vi "log analysis_gps.vi"() -> ()   [LabVIEW 2018] (continued)
\t0.279000\t0.031000\n\t\n15:35:17.6\tlog_raw\tgps_raw\t#DUALANTENNAHEADINGA,USB3,0,49.5,FINESTEERING,2107,282935.600,02000000,d426,15824;INSUFFICIENT_OBS,NONE,-1.000000000,0.000000000,0.000000000,0.0,0.000000000,0.000000000,\"631T\",15,2,2,2,04,00,20,00*646f005d\n\tsystem status\tnormal 2 28.000000 0 0\trobot status\t256.780314\t90.298273\t8.714600\t-0.760632\t-2.225127\t150.467339\t0.388000\t-0.122000\n\t\n15:35:18.1\tlog_raw\tgps_raw\t#DUALANTENNAHEADINGA,USB3,0,49.5,FINESTEERING,2107,282936.100,02000000,d426,15824;INSUFFICIENT_OBS,NONE,-1.000000000,0.000000000,0.000000000,0.0,0.000000000,0.000000000,\"631T\",15,2,2,2,04,00,20,00*1eaf17a0\n\tsystem status\tnormal 2 27.900000 0 0\trobot status\t256.663990\t90.379029\t8.710300\t-0.683394\t-2.214514\t150.522988\t0.256000\t0.072000\n\t\n15:35:18.6\tlog_raw\tgps_raw\t#DUALANTENNAHEADINGA,USB3,0,49.5,FINESTEERING,2107,282936.600,02000000,d426,15824;INSUFFICIENT_OBS,NONE,-1.000000000,0.000000000,0.000000000,0.0,0.000000000,0.000000000,\"631T\",15,2,2,2,04,00,20,00*d2070d36\n\tsystem status\tnormal 2 28.000000 0 0\trobot status\t256.545030\t90.462138\t8.705100\t-0.490639\t-2.202791\t150.542142\t0.254000\t0.061000\n\t\n15:35:19.1\tlog_raw\tgps_raw\t#DUALANTENNAHEADINGA,USB3,0,49.5,FINESTEERING,2107,282937.100,02000000,d426,15824;INSUFFICIENT_OBS,NONE,-1.000000000,0.000000000,0.000000000,0.0,0.000000000,0.000000000,\"631T\",15,2,2,2,04,00,20,00*73771379\n\tsystem status\tnormal 2 27.900000 0 0\trobot status\t256.425827\t90.542953\t8.700000\t-0.567939\t-2.228448\t150.645686\t0.243000\t0.082000\n\t\n15:35:19.6\tlog_raw\tgps_raw\t#DUALANTENNAHEADINGA,USB3,0,50.0,FINESTEERING,2107,282937.600,02000000,d426,15824;INSUFFICIENT_OBS,NONE,-1.000000000,0.000000000,0.000000000,0.0,0.000000000,0.000000000,\"631T\",16,2,2,2,04,00,20,00*68ac25ab\n\tsystem status\tnormal 2 27.900000 0 0\trobot status\t256.306306\t90.622871\t8.696700\t-0.661354\t-2.128158\t150.731139\t0.241000\t0.099000\n\t\n15:35:20.1\tlog_raw\tgps_raw\t#DUALANTENNAHEADINGA,USB3,0,50.0,FINESTEERING,2107,282938.100,02000000,d426,15824;INSUFFICIENT_OBS,NONE,-1.000000000,0.000000000,0.000000000,0.0,0.000000000,0.000000000,\"631T\",16,2,2,2,04,00,20,00*a65f0d39\n\tsystem status\tnormal 2 27.900000 0 0\trobot status\t256.186382\t90.704627\t8.692700\t-0.606127\t-2.269498\t150.834524\t0.254000\t0.081000\n\t\n15:35:20.6\tlog_raw\tgps_raw\t#DUALANTENNAHEADINGA,USB3,0,50.0,FINESTEERING,2107,282938.600,02000000,d426,15824;INSUFFICIENT_OBS,NONE,-1.000000000,0.000000000,0.000000000,0.0,0.000000000,0.000000000,\"631T\",17,2,2,2,04,00,20,00*bd1597f7\n\tsystem status\tnormal 2 27.900000 0 0\trobot status\t256.067025\t90.786079\t8.688900\t-0.322241\t-2.499892\t151.028878\t0.352000\t-0.085000\n\t\n15:35:21.1\tlog_raw\tgps_raw\t#DUALANTENNAHEADINGA,USB3,0,50.0,FINESTEERING,2107,282939.100,02000000,d426,15824;INSUFFICIENT_OBS,NONE,-1.000000000,0.000000000,0.000000000,0.0,0.000000000,0.000000000,\"631T\",17,2,2,2,04,00,20,00*1c6589b8\n\tsystem status\tnormal 2 28.000000 0 0\trobot status\t255.947562\t90.865503\t8.685500\t-0.303833\t-2.363936\t151.114565\t0.300000\t0.000000\n\t\n15:35:21.6\tlog_raw\tgps_raw\t#DUALANTENNAHEADINGA,USB3,0,52.0,FINESTEERING,2107,282939.600,02000000,d426,15824;INSUFFICIENT_OBS,NONE,-1.000000000,0.000000000,0.000000000,0.0,0.000000000,0.000000000,\"631T\",14,2,2,2,04,00,20,00*bb12b8cf\n\tsystem status\tnormal 2 27.900000 0 0\trobot status\t255.828620\t90.941630\t8.682600\t-0.556904\t-2.247705\t151.117171\t0.272000\t0.029000\n\t\n15:35:22.1\tlog_raw\tgps_raw\t#DUALANTENNAHEADINGA,USB3,0,50.0,FINESTEERING,2107,282940.100,02000000,d426,15824;INSUFFICIENT_OBS,NONE,-1.000000000,0.000000000,0.000000000,0.0,0.000000000,0.000000000,\"631T\",14,2,2,2,04,00,20,00*9b77340d\n\tsystem status\tnormal 2 27.900000 0 0\trobot status\t255.707606\t91.021162\t8.679300\t-0.530900\t-2.252938\t151.145444\t0.328000\t-0.057000\n\t\n15:35:22.6\tlog_raw\tgps_raw\t#INSPVAXA,USB3,0,50.0,FINESTEERING,2107,282940.600,02000000,471d,15824;INS_ALIGNMENT_COMPLETE,INS_RTKFIXED,37.37095109367,126.72372052515,8.6731,22.3000,0.1517,-0.2300,-0.0234,-0.267173329,-2.329530247,298.720230899,0.4406,0.2945,0.5541,0.1133,0.0925,0.0773,0.0978,0.1028,4.9197,0f000001,0*f2292127\n\tsystem status\tnormal 2 28.000000 0 0\trobot status\t255.585782\t91.103037\t8.673100\t-0.267173\t-2.329530\t151.279769\t0.419000\t-0.188000\n\t\n15:35:23.1\tlog_raw\tgps_raw\t#DUALANTENNAHEADINGA,USB3,0,49.5,FINESTEERING,2107,282941.100,02000000,d426,15824;INSUFFICIENT_OBS,NONE,-1.000000000,0.000000000,0.000000000,0.0,0.000000000,0.000000000,\"631T\",17,2,2,2,04,00,20,00*21dc1c90\n\tsystem status\tnormal 2 28.000000 0 0\trobot status\t255.466813\t91.182906\t8.667600\t-0.154589\t-2.350516\t151.330010\t0.342000\t-0.053000\n\t\n15:35:23.6\tlog_raw\tgps_raw\t#DUALANTENNAHEADINGA,USB3,0,49.5,FINESTEERING,2107,282941.600,02000000,d426,15824;INSUFFICIENT_OBS,NONE,-1.000000000,0.000000000,0.000000000,0.0,0.000000000,0.000000000,\"631T\",17,2,2,2,04,00,20,00*ed740606\n\tsystem status\tnormal 2 28.000000 0 0\trobot status\t255.348341\t91.260716\t8.663400\t-0.359685\t-2.297097\t151.358113\t0.271000\t0.037000\n\t\n15:35:24.1\tlog_raw\tgps_raw\t#DUALANTENNAHEADINGA,USB3,0,49.5,FINESTEERING,2107,282942.100,02000000,d426,15824;INSUFFICIENT_OBS,NONE,-1.000000000,0.000000000,0.000000000,0.0,0.000000000,0.000000000,\"631T\",15,2,2,2,04,00,20,00*e300170a\n\tsystem status\tnormal 2 27.900000 0 0\trobot status\t255.227088\t91.341470\t8.659200\t-0.418788\t-2.494250\t151.398248\t0.269000\t0.061000\n\t\n15:35:24.6\tlog_raw\tgps_raw\t#DUALANTENNAHEADINGA,USB3,0,49.5,FINESTEERING,2107,282942.600,02000000,d426,15824;INSUFFICIENT_OBS,NONE,-1.000000000,0.000000000,0.000000000,0.0,0.000000000,0.000000000,\"631T\",13,2,2,2,04,00,20,00*b274068f\n\tsystem status\tnormal 2 28.000000 0 0\trobot status\t255.107667\t91.421781\t8.652400\t-0.280884\t-2.457147\t151.424820\t0.260000\t0.059000\n\t\n15:35:25.1\tlog_raw\tgps_raw\t#DUALANTENNAHEADINGA,USB3,0,49.5,FINESTEERING,2107,282943.100,02008000,d426,15824;INSUFFICIENT_OBS,NONE,-1.000000000,0.000000000,0.000000000,0.0,0.000000000,0.000000000,\"631T\",13,2,2,2,04,00,20,00*05979c61\n\tsystem status\tnormal 2 28.000000 0 0\trobot status\t254.990314\t91.500800\t8.645200\t-0.235303\t-2.314324\t151.467138\t0.287000\t0.019000\n\t\n15:35:25.6\tlog_raw\tgps_raw\t#DUALANTENNAHEADINGA,USB3,0,50.0,FINESTEERING,2107,282943.600,02008000,d426,15824;INSUFFICIENT_OBS,NONE,-1.000000000,0.000000000,0.000000000,0.0,0.000000000,0.000000000,\"631T\",15,2,2,2,04,00,20,00*20c62709\n\tsystem status\tnormal 2 28.000000 0 0\trobot status\t254.870895\t91.580665\t8.639100\t-0.192889\t-2.377459\t151.460910\t0.281000\t0.026000\n\t\n15:35:26.1\tlog_raw\tgps_raw\t#DUALANTENNAHEADINGA,USB3,0,50.0,FINESTEERING,2107,282944.100,02008000,d426,15824;INSUFFICIENT_OBS,NONE,-1.000000000,0.000000000,0.000000000,0.0,0.000000000,0.000000000,\"631T\",15,2,2,2,04,00,20,00*361725d1\n\tsystem status\tnormal 2 28.000000 0 0\trobot status\t254.750757\t91.660864\t8.633300\t-0.180871\t-2.554639\t151.458844\t0.261000\t0.067000\n\t\n15:35:26.6\tlog_raw\tgps_raw\t#DUALANTENNAHEADINGA,USB3,0,53.0,FINESTEERING,2107,282944.600,02008000,d426,15824;INSUFFICIENT_OBS,NONE,-1.000000000,0.000000000,0.000000000,0.0,0.000000000,0.000000000,\"631T\",15,2,2,2,04,00,20,00*567244ab\n\tsystem status\tnormal 2 28.000000 0 0\trobot status\t254.630389\t91.742058\t8.625500\t-0.192952\t-2.590747\t151.439255\t0.283000\t0.030000\n\t\n15:35:27.1\tlog_raw\tgps_raw\t#DUALANTENNAHEADINGA,USB3,0,52.5,FINESTEERING,2107,282945.100,02008000,d426,15824;INSUFFICIENT_OBS,NONE,-1.000000000,0.000000000,0.000000000,0.0,0.000000000,0.000000000,\"631T\",13,2,2,2,04,00,20,00*5be0619f\n\tsystem status\tnormal 2 28.000000 0 0\trobot status\t254.513468\t91.822238\t8.617100\t-0.159086\t-2.547197\t151.443587\t0.276000\t0.035000\n\t\n15:35:27.6\tlog_raw\tgps_raw\t#DUALANTENNAHEADINGA,USB3,0,52.5,FINESTEERING,2107,282945.600,02008000,d426,15824;INSUFFICIENT_OBS,NONE,-1.000000000,0.000000000,0.000000000,0.0,0.000000000,0.000000000,\"631T\",13,2,2,2,04,00,20,00*97487b09\n\tsystem status\tnormal 2 28.000000 0 0\trobot status\t254.392942\t91.902806\t8.609000\t-0.121394\t-2.673746\t151.420849\t0.277000\t0.034000\n\t\n15:35:28.1\tlog_raw\tgps_raw\t#DUALANTENNAHEADINGA,USB3,0,49.5,FINESTEERING,2107,282946.100,02008000,d426,15824;INSUFFICIENT_OBS,NONE,-1.000000000,0.000000000,0.000000000,0.0,0.000000000,0.000000000,\"631T\",14,2,2,2,04,00,20,00*4e6006d6\n\tsystem status\tnormal 2 28.000000 0 0\trobot status\t254.275148\t91.981980\t8.600700\t-0.137266\t-2.581289\t151.414534\t0.312000\t-0.003000\n\t\n15:35:28.6\tlog_raw\tgps_raw\t#DUALANTENNAHEADINGA,USB3,0,49.5,FINESTEERING,2107,282946.600,02008000,d426,15824;INSUFFICIENT_OBS,NONE,-1.000000000,0.000000000,0.000000000,0.0,0.000000000,0.000000000,\"631T\",15,2,2,2,04,00,20,00*552a9c18\n\tsystem status\tnormal 2 28.000000 0 0\trobot status\t254.158680\t92.060277\t8.593000\t-0.236334\t-2.525811\t151.415418\t0.436000\t-0.193000\n\t\n15:35:29.1\tlog_raw\tgps_raw\t#DUALANTENNAHEADINGA,USB3,0,48.5,FINESTEERING,2107,282947.100,02008000,d426,15824;INSUFFICIENT_OBS,NONE,-1.000000000,0.000000000,0.000000000,0.0,0.000000000,0.000000000,\"631T\",16,2,2,2,04,00,20,00*3348d25a\n\tsystem status\tnormal 2 28.000000 0 0\trobot status\t254.042373\t92.139923\t8.584700\t-0.240278\t-2.555508\t151.434704\t0.283000\t0.033000\n\t\n15:35:29.6\tlog_raw\tgps_raw\t#DUALANTENNAHEADINGA,USB3,0,48.5,FINESTEERING,2107,282947.600,02000000,d426,15824;INSUFFICIENT_OBS,NONE,-1.000000000,0.000000000,0.000000000,0.0,0.000000000,0.000000000,\"631T\",16,2,2,2,04,00,20,00*e9734c6d\n\tsystem status\tnormal 2 27.900000 0 0\trobot status\t253.922648\t92.221882\t8.576200\t-0.258547\t-2.691459\t151.424743\t0.237000\t0.095000\n\t\n15:35:30.1\tlog_raw\tgps_raw\t#DUALANTENNAHEADINGA,USB3,0,48.5,FINESTEERING,2107,282948.100,02000000,d426,15824;INSUFFICIENT_OBS,NONE,-1.000000000,0.000000000,0.000000000,0.0,0.000000000,0.000000000,\"631T\",16,2,2,2,04,00,20,00*278064ff\n\tsystem status\tnormal 2 28.000000 0 0\trobot status\t253.805920\t92.302649\t8.568900\t-0.289763\t-2.670093\t151.392243\t0.351000\t-0.076000\n\t\n15:35:30.6\tlog_raw\tgps_raw\t#DUALANTENNAHEADINGA,USB3,0,49.0,FINESTEERING,2107,282948.600,02000000,d426,15824;INSUFFICIENT_OBS,NONE,-1.000000000,0.000000000,0.000000000,0.0,0.000000000,0.000000000,\"631T\",16,2,2,2,04,00,20,00*da164e01\n\tsystem status\tnormal 2 28.000000 0 0\trobot status\t253.687845\t92.382279\t8.561200\t-0.417432\t-2.808123\t151.452850\t0.423000\t-0.185000\n\t\n15:35:31.1\tlog_raw\tgps_raw\t#DUALANTENNAHEADINGA,USB3,0,49.0,FINESTEERING,2107,282949.100,02008000,d426,15824;INSUFFICIENT_OBS,NONE,-1.000000000,0.000000000,0.000000000,0.0,0.000000000,0.000000000,\"631T\",16,2,2,2,04,00,20,00*6df5d4ef\n\tsystem status\tnormal 2 27.900000 0 0\trobot status\t253.568870\t92.461854\t8.552900\t-0.517935\t-2.852279\t151.503432\t0.247000\t0.081000\n\t\n15:35:31.6\tlog_raw\tgps_raw\t#DUALANTENNAHEADINGA,USB3,0,50.5,FINESTEERING,2107,282949.600,02008000,d426,15824;INSUFFICIENT_OBS,NONE,-1.000000000,0.000000000,0.000000000,0.0,0.000000000,0.000000000,\"631T\",16,2,2,2,04,00,20,00*d5786494\n\tsystem status\tnormal 2 27.900000 0 0\trobot status\t253.447549\t92.540563\t8.545300\t-0.634770\t-2.802068\t151.569225\t0.458000\t-0.230000\n\t\n15:35:32.1\tlog_raw\tgps_raw\t#DUALANTENNAHEADINGA,USB3,0,50.5,FINESTEERING,2107,282950.100,02008000,d426,15824;INSUFFICIENT_OBS,NONE,-1.000000000,0.000000000,0.000000000,0.0,0.000000000,0.000000000,\"631T\",16,2,2,2,04,00,20,00*5348e2e5\n\tsystem status\tnormal 2 28.000000 0 0\trobot status\t253.327603\t92.619270\t8.538000\t-0.695995\t-2.872123\t151.658329\t0.256000\t0.081000\n\t\n15:35:32.6\tlog_raw\tgps_raw\t#DUALANTENNAHEADINGA,USB3,0,50.5,FINESTEERING,2107,282950.600,02008000,d426,15824;INSUFFICIENT_OBS,NONE,-1.000000000,0.000000000,0.000000000,0.0,0.000000000,0.000000000,\"631T\",16,2,2,2,04,00,20,00*9fe0f873\n\tsystem status\tnormal 2 27.900000 0 0\trobot status\t253.206959\t92.699516\t8.530600\t-0.579326\t-2.998121\t151.745125\t0.276000\t0.032000\n\t\n15:35:33.1\tlog_raw\tgps_raw\t#DUALANTENNAHEADINGA,USB3,0,48.0,FINESTEERING,2107,282951.100,02008000,d426,15824;INSUFFICIENT_OBS,NONE,-1.000000000,0.000000000,0.000000000,0.0,0.000000000,0.000000000,\"631T\",16,2,2,2,04,00,20,00*2ef19a75\n\tsystem status\tnormal 2 27.900000 0 0\trobot status\t253.086641\t92.778208\t8.522800\t-0.669072\t-2.968137\t151.793358\t0.305000\t-0.020000\n\t\n15:35:33.6\tlog_raw\tgps_raw\t#DUALANTENNAHEADINGA,USB3,0,48.0,FINESTEERING,2107,282951.600,02008000,d426,15824;INSUFFICIENT_OBS,NONE,-1.000000000,0.000000000,0.000000000,0.0,0.000000000,0.000000000,\"631T\",17,2,2,2,04,00,20,00*35bb00bb\n\tsystem status\tnormal 2 28.000000 0 0\trobot status\t252.966146\t92.856684\t8.515700\t-0.823336\t-2.969880\t151.842849\t0.277000\t0.026000\n\t\n15:35:34.1\tlog_raw\tgps_raw\t\tsystem status\tnormal 2 27.900000 0 0\trobot status\t252.845707\t92.935485\t8.508700\t-0.946775\t-3.084704\t151.928566\t0.199000\t0.137000\n\t\n15:35:34.6\tlog_raw\tgps_raw\t\tsystem status\tnormal 2 28.000000 0 0\trobot status\t252.727118\t93.014271\t8.504100\t-0.880224\t-2.934570\t152.110413\t0.448000\t-0.238000\n\t\n15:35:35.1\tlog_raw\tgps_raw\t#DUALANTENNAHEADINGA,USB3,0,47.5,FINESTEERING,2107,282953.100,02008000,d426,15824;INSUFFICIENT_OBS,NONE,-1.000000000,0.000000000,0.000000000,0.0,0.000000000,0.000000000,\"631T\",14,2,2,2,04,00,20,00*a6e4ed65\n\tsystem status\tnormal 2 27.900000 0 0\trobot status\t252.606768\t93.093325\t8.499800\t-0.892042\t-2.837254\t152.160427\t0.275000\t0.033000\n\t\n15:35:35.6\tlog_raw\tgps_raw\t#DUALANTENNAHEADINGA,USB3,0,50.0,FINESTEERING,2107,282953.600,02000000,d426,15824;INSUFFICIENT_OBS,NONE,-1.000000000,0.000000000,0.000000000,0.0,0.000000000,0.000000000,\"631T\",13,2,2,2,04,00,20,00*54eb1acf\n\tsystem status\tnormal 2 27.900000 0 0\trobot status\t252.486962\t93.170128\t8.495600\t-0.968428\t-2.739285\t152.198894\t0.348000\t-0.080000\n\t\n15:35:36.1\tlog_raw\tgps_raw\t#DUALANTENNAHEADINGA,USB3,0,48.0,FINESTEERING,2107,282954.100,02000000,d426,15824;INSUFFICIENT_OBS,NONE,-1.000000000,0.000000000,0.000000000,0.0,0.000000000,0.000000000,\"631T\",14,2,2,2,04,00,20,00*4d1f09d9\n\tsystem status\tnormal 2 27.900000 0 0\trobot status\t252.367322\t93.248054\t8.491100\t-0.955023\t-2.515838\t152.247418\t0.357000\t-0.086000\n\t\n15:35:36.6\tlog_raw\tgps_raw\t#DUALANTENNAHEADINGA,USB3,0,48.0,FINESTEERING,2107,282954.600,02000000,d426,15824;INSUFFICIENT_OBS,NONE,-1.000000000,0.000000000,0.000000000,0.0,0.000000000,0.000000000,\"631T\",16,2,2,2,04,00,20,00*f50315be\n\tsystem status\tnormal 2 28.000000 0 0\trobot status\t252.247855\t93.326149\t8.487100\t-0.842888\t-2.348222\t152.261330\t0.322000\t-0.041000\n\t\n15:35:37.1\tlog_raw\tgps_raw\t#INSPVAXA,USB3,0,47.5,FINESTEERING,2107,282955.150,02000000,471d,15824;INS_ALIGNMENT_COMPLETE,INS_RTKFIXED,37.37097191028,126.72368135449,8.4841,22.3000,0.1693,-0.2422,-0.0142,-0.799407397,-2.166438439,297.747094152,0.4450,0.2953,0.5584,0.1141,0.0928,0.0775,0.0978,0.1030,4.9299,0f000001,0*711ec271\n\tsystem status\tnormal 2 28.000000 0 0\trobot status\t252.116109\t93.413465\t8.484100\t-0.799407\t-2.166438\t152.252906\t0.332000\t-0.052000\n\t\n15:35:37.6\tlog_raw\tgps_raw\t#DUALANTENNAHEADINGA,USB3,0,47.5,FINESTEERING,2107,282955.600,02000000,d426,15824;INSUFFICIENT_OBS,NONE,-1.000000000,0.000000000,0.000000000,0.0,0.000000000,0.000000000,\"631T\",13,2,2,2,04,00,20,00*8140e48e\n\tsystem status\tnormal 2 27.900000 0 0\trobot status\t252.011078\t93.483113\t8.481000\t-0.846538\t-1.955023\t152.315960\t0.339000\t-0.062000\n\t\n15:35:38.1\tlog_raw\tgps_raw\t#DUALANTENNAHEADINGA,USB3,0,47.5,FINESTEERING,2107,282956.100,02000000,d426,15824;INSUFFICIENT_OBS,NONE,-1.000000000,0.000000000,0.000000000,0.0,0.000000000,0.000000000,\"631T\",14,2,2,2,04,00,20,00*b1be7838\n\tsystem status\tnormal 2 27.900000 0 0\trobot status\t251.892792\t93.560878\t8.478700\t-1.086649\t-1.737827\t152.384884\t0.296000\t-0.002000\n\t\n15:35:38.6\tlog_raw\tgps_raw\t\tsystem status\tnormal 2 28.000000 0 0\trobot status\t251.773181\t93.640986\t8.476600\t-0.964983\t-1.456887\t152.427884\t0.357000\t-0.090000\n\t\n15:35:39.1\tlog_raw\tgps_raw\t#DUALANTENNAHEADINGA,USB3,0,49.5,FINESTEERING,2107,282957.100,02000000,d426,15824;INSUFFICIENT_OBS,NONE,-1.000000000,0.000000000,0.000000000,0.0,0.000000000,0.000000000,\"631T\",15,2,2,2,04,00,20,00*1dabb482\n\tsystem status\tnormal 2 28.000000 0 0\trobot status\t251.654659\t93.722946\t8.475100\t-0.668177\t-1.430088\t152.409420\t0.366000\t-0.112000\n\t\n15:35:39.6\tlog_raw\tgps_raw\t\tsystem status\tnormal 2 28.000000 0 0\trobot status\t251.542323\t93.800199\t8.475200\t-0.574923\t-1.096038\t152.514245\t0.289000\t-0.013000\n\t\n15:35:40.1\tlog_raw\tgps_raw\t#DUALANTENNAHEADINGA,USB3,0,47.5,FINESTEERING,2107,282958.100,02000000,d426,15824;INSUFFICIENT_OBS,NONE,-1.000000000,0.000000000,0.000000000,0.0,0.000000000,0.000000000,\"631T\",14,2,2,2,04,00,20,00*de3d4ee5\n\tsystem status\tnormal 2 28.000000 0 0\trobot status\t251.415981\t93.883006\t8.474100\t-0.824722\t-1.034335\t152.447929\t0.230000\t0.080000\n\t\n15:35:40.6\tlog_raw\tgps_raw\t#DUALANTENNAHEADINGA,USB3,0,47.5,FINESTEERING,2107,282958.600,02000000,d426,15824;INSUFFICIENT_OBS,NONE,-1.000000000,0.000000000,0.000000000,0.0,0.000000000,0.000000000,\"631T\",15,2,2,2,04,00,20,00*c577d42b\n\tsystem status\tnormal 2 28.000000 0 0\trobot status\t251.291310\t93.963969\t8.471000\t-1.101436\t-1.443310\t152.459219\t0.236000\t0.098000\n\t\n15:35:41.1\tlog_raw\tgps_raw\t#DUALANTENNAHEADINGA,USB3,0,47.5,FINESTEERING,2107,282959.100,02000000,d426,15824;INSUFFICIENT_OBS,NONE,-1.000000000,0.000000000,0.000000000,0.0,0.000000000,0.000000000,\"631T\",15,2,2,2,04,00,20,00*6407ca64\n\tsystem status\tnormal 2 28.000000 0 0\trobot status\t251.172018\t94.044368\t8.468600\t-1.020791\t-1.480021\t152.538410\t0.271000\t0.040000\n\t\n15:35:41.6\tlog_raw\tgps_raw\t#INSPVAXA,USB3,0,50.5,FINESTEERING,2107,282959.650,02000000,471d,15824;INS_ALIGNMENT_COMPLETE,INS_RTKFIXED,37.37097835365,126.72366921356,8.4679,22.3000,0.1677,-0.2288,-0.0117,-1.228660842,-1.304176220,297.349897082,0.4459,0.2954,0.5577,0.1140,0.0926,0.0775,0.0977,0.1029,4.9210,0f000001,0*0060fe10\n\tsystem status\tnormal 2 27.900000 0 0\trobot status\t251.040686\t94.128612\t8.467900\t-1.228661\t-1.304176\t152.650103\t0.294000\t0.025000\n\t\n15:35:42.1\tlog_raw\tgps_raw\t#DUALANTENNAHEADINGA,USB3,0,50.5,FINESTEERING,2107,282960.100,02000000,d426,15824;INSUFFICIENT_OBS,NONE,-1.000000000,0.000000000,0.000000000,0.0,0.000000000,0.000000000,\"631T\",15,2,2,2,04,00,20,00*3c5b3030\n\tsystem status\tnormal 2 27.900000 0 0\trobot status\t250.933323\t94.199664\t8.470400\t-1.218748\t-1.601096\t152.690711\t0.293000\t0.046000\n\t\n15:35:42.6\tlog_raw\tgps_raw\t#INSPVAXA,USB3,0,51.0,FINESTEERING,2107,282960.650,02000000,471d,15824;INS_ALIGNMENT_COMPLETE,INS_RTKFIXED,37.37097975694,126.72366653039,8.4696,22.3000,0.1798,-0.2500,-0.0237,-1.216813697,-1.020291327,297.186745647,0.4456,0.2953,0.5575,0.1139,0.0925,0.0775,0.0977,0.1029,4.9186,0f000001,0*5a2daee3\n\tsystem status\tnormal 2 27.900000 0 0\trobot status\t250.803015\t94.284363\t8.469600\t-1.216814\t-1.020291\t152.813254\t0.376000\t-0.091000\n\t\n15:35:43.1\tlog_raw\tgps_raw\t#INSPVAXA,USB3,0,49.5,FINESTEERING,2107,282961.150,02000000,471d,15824;INS_ALIGNMENT_COMPLETE,INS_RTKFIXED,37.37098043030,126.72366522949,8.4707,22.3000,0.1736,-0.2321,-0.0202,-1.283284978,-0.599057557,297.054686065,0.4445,0.2952,0.5571,0.1143,0.0927,0.0774,0.0977,0.1029,4.9180,0f000001,0*2a0011a7\n\tsystem status\tnormal 2 27.900000 0 0\trobot status\t250.687783\t94.359099\t8.470700\t-1.283285\t-0.599058\t152.945314\t0.285000\t0.038000\n\t\n15:35:43.6\tlog_raw\tgps_raw\t#INSPVAXA,USB3,0,49.5,FINESTEERING,2107,282961.650,02000000,471d,15824;INS_ALIGNMENT_COMPLETE,INS_RTKFIXED,37.37098110598,126.72366388035,8.4719,22.3000,0.1770,-0.2280,-0.0121,-1.256734813,-0.468526874,296.976116975,0.4445,0.2952,0.5571,0.1143,0.0927,0.0774,0.0977,0.1029,4.9180,0f000001,0*1df4362b\n\tsystem status\tnormal 2 27.900000 0 0\trobot status\t250.568279\t94.434093\t8.471900\t-1.256735\t-0.468527\t153.023883\t0.258000\t0.074000\n\t\n15:35:44.1\tlog_raw\tgps_raw\t\tsystem status\tnormal 2 27.900000 0 0\trobot status\t250.460513\t94.502707\t8.473000\t-1.216741\t-0.450959\t153.062982\t0.253000\t0.073000\n\t\n15:35:44.6\tlog_raw\tgps_raw\t#INSPVAXA,USB3,0,47.5,FINESTEERING,2107,282962.650,02000000,471d,15824;INS_ALIGNMENT_COMPLETE,INS_RTKFIXED,37.37098248042,126.72366115831,8.4743,22.3000,0.1748,-0.2259,-0.0058,-1.109471355,-0.449070026,296.783460113,0.4449,0.2952,0.5570,0.1145,0.0926,0.0774,0.0977,0.1028,4.9165,0f000001,0*1baf4086\n\tsystem status\tnormal 2 27.900000 0 0\trobot status\t250.327165\t94.586642\t8.474300\t-1.109471\t-0.449070\t153.216540\t0.253000\t0.063000\n\t\n15:35:45.1\tlog_raw\tgps_raw\t#INSPVAXA,USB3,0,50.0,FINESTEERING,2107,282963.150,02000000,471d,15824;INS_ALIGNMENT_COMPLETE,INS_RTKFIXED,37.37098316293,126.72365977185,8.4754,22.3000,0.1768,-0.2291,-0.0058,-1.166384904,-0.522599748,296.670399904,0.4455,0.2951,0.5568,0.1141,0.0925,0.0774,0.0977,0.1028,4.9146,0f000001,0*0f185e23\n\tsystem status\tnormal 2 27.900000 0 0\trobot status\t250.204354\t94.662394\t8.475400\t-1.166385\t-0.522600\t153.329600\t0.333000\t-0.037000\n\t\n15:35:45.6\tlog_raw\tgps_raw\t#INSPVAXA,USB3,0,50.0,FINESTEERING,2107,282963.650,02000000,471d,15824;INS_ALIGNMENT_COMPLETE,INS_RTKFIXED,37.37098384842,126.72365839732,8.4765,22.3000,0.1700,-0.2283,-0.0073,-1.035044239,-0.558854853,296.631402056,0.4455,0.2951,0.5568,0.1141,0.0925,0.0774,0.0977,0.1028,4.9146,0f000001,0*d0797a7e\n\tsystem status\tnormal 2 27.900000 0 0\trobot status\t250.082601\t94.738476\t8.476500\t-1.035044\t-0.558855\t153.368598\t0.256000\t0.071000\n\t\n15:35:46.1\tlog_raw\tgps_raw\t#INSPVAXA,USB3,0,47.5,FINESTEERING,2107,282964.150,02000000,471d,15824;INS_ALIGNMENT_COMPLETE,INS_RTKFIXED,37.37098452995,126.72365703977,8.4774,22.3000,0.1687,-0.2278,-0.0051,-0.825749574,-0.403704202,296.577547873,0.4447,0.2949,0.5563,0.1141,0.0926,0.0774,0.0977,0.1028,4.9134,0f000001,0*96a6dd12\n\tsystem status\tnormal 2 28.000000 0 0\trobot status\t249.962351\t94.814119\t8.477400\t-0.825750\t-0.403704\t153.422452\t0.285000\t0.028000\n\t\n15:35:46.6\tlog_raw\tgps_raw\t#DUALANTENNAHEADINGA,USB3,0,47.5,FINESTEERING,2107,282964.600,02000000,d426,15824;INSUFFICIENT_OBS,NONE,-1.000000000,0.000000000,0.000000000,0.0,0.000000000,0.000000000,\"631T\",13,2,2,2,04,00,20,00*364e308a\n\tsystem status\tnormal 2 27.900000 0 0\trobot status\t249.853356\t94.880309\t8.477500\t-0.801435\t-0.341855\t153.481008\t0.370000\t-0.101000\n\t\n15:35:47.1\tlog_raw\tgps_raw\t#INSPVAXA,USB3,0,49.0,FINESTEERING,2107,282965.150,02000000,471d,15824;INS_ALIGNMENT_COMPLETE,INS_RTKFIXED,37.37098586278,126.72365430292,8.4776,22.3000,0.1652,-0.2280,-0.0084,-0.812912729,-0.298745474,296.545314243,0.4441,0.2948,0.5560,0.1139,0.0926,0.0774,0.0977,0.1027,4.9127,0f000001,0*10118c42\n\tsystem status\tnormal 2 28.000000 0 0\trobot status\t249.719925\t94.962050\t8.477600\t-0.812913\t-0.298745\t153.454686\t0.258000\t0.063000\n\t\n15:35:47.6\tlog_raw\tgps_raw\t#INSPVAXA,USB3,0,49.0,FINESTEERING,2107,282965.650,02000000,471d,15824;INS_ALIGNMENT_COMPLETE,INS_RTKFIXED,37.37098653582,126.72365294600,8.4789,22.3000,0.1677,-0.2410,-0.0069,-0.826772315,0.019774028,296.533621438,0.4441,0.2948,0.5560,0.1139,0.0926,0.0774,0.0977,0.1027,4.9127,0f000001,0*1d42ccbf\n\tsystem status\tnormal 2 28.000000 0 0\trobot status\t249.599732\t95.036751\t8.478900\t-0.826772\t0.019774\t153.466379\t0.367000\t-0.093000\n\t\n15:35:48.1\tlog_raw\tgps_raw\t\tsystem status\tnormal 2 27.900000 0 0\trobot status\t249.492164\t95.103838\t8.479600\t-0.859418\t0.051260\t153.510100\t0.350000\t-0.075000\n\t\n15:35:48.6\tlog_raw\tgps_raw\t\tsystem status\tnormal 2 28.000000 0 0\trobot status\t249.368260\t95.179421\t8.479400\t-0.924661\t-0.189774\t153.513644\t0.248000\t0.068000\n\t\n15:35:49.1\tlog_raw\tgps_raw\t#DUALANTENNAHEADINGA,USB3,0,48.5,FINESTEERING,2107,282967.100,02000000,d426,15824;INSUFFICIENT_OBS,NONE,-1.000000000,0.000000000,0.000000000,0.0,0.000000000,0.000000000,\"631T\",13,2,2,2,04,00,20,00*3ee5b9e8\n\tsystem status\tnormal 2 28.000000 0 0\trobot status\t249.246534\t95.255236\t8.479300\t-0.943512\t-0.176843\t153.495660\t0.260000\t0.060000\n\t\n15:35:49.6\tlog_raw\tgps_raw\t#INSPVAXA,USB3,0,48.5,FINESTEERING,2107,282967.650,02000000,471d,15824;INS_ALIGNMENT_COMPLETE,INS_RTKFIXED,37.37098925178,126.72364742874,8.4811,22.3000,0.1700,-0.2499,-0.0176,-0.986615151,-0.569191402,296.569428788,0.4450,0.2948,0.5562,0.1138,0.0925,0.0774,0.0977,0.1027,4.9114,0f000001,0*8120b203\n\tsystem status\tnormal 2 28.000000 0 0\trobot status\t249.111022\t95.338195\t8.481100\t-0.986615\t-0.569191\t153.430571\t0.300000\t0.000000\n\t\n15:35:50.1\tlog_raw\tgps_raw\t#INSPVAXA,USB3,0,51.0,FINESTEERING,2107,282968.150,02000000,471d,15824;INS_ALIGNMENT_COMPLETE,INS_RTKFIXED,37.37098994015,126.72364604242,8.4821,22.3000,0.1610,-0.2295,-0.0122,-1.022493310,-0.855866678,296.640582701,0.4448,0.2947,0.5563,0.1137,0.0927,0.0774,0.0977,0.1027,4.9112,0f000001,0*d8f4721a\n\tsystem status\tnormal 2 28.000000 0 0\trobot status\t248.988224\t95.414597\t8.482100\t-1.022493\t-0.855867\t153.359417\t0.284000\t0.007000\n\t\n15:35:50.6\tlog_raw\tgps_raw\t#INSPVAXA,USB3,0,51.0,FINESTEERING,2107,282968.650,02000000,471d,15824;INS_ALIGNMENT_COMPLETE,INS_RTKFIXED,37.37099061783,126.72364467060,8.4818,22.3000,0.1613,-0.2282,-0.0121,-1.153302728,-0.788505440,296.737399277,0.4448,0.2947,0.5563,0.1137,0.0927,0.0774,0.0977,0.1027,4.9112,0f000001,0*561016f0\n\tsystem status\tnormal 2 28.000000 0 0\trobot status\t248.866710\t95.489813\t8.481800\t-1.153303\t-0.788505\t153.262601\t0.294000\t0.000000\n\t\n15:35:51.1\tlog_raw\tgps_raw\t#INSPVAXA,USB3,0,51.0,FINESTEERING,2107,282969.150,02000000,471d,15824;INS_ALIGNMENT_COMPLETE,INS_RTKFIXED,37.37099130336,126.72364331886,8.4815,22.3000,0.1682,-0.2376,-0.0147,-1.125512606,-0.794604526,296.797111789,0.4434,0.2946,0.5560,0.1136,0.0926,0.0774,0.0977,0.1027,4.9114,0f000001,0*989702a1\n\tsystem status\tnormal 2 28.000000 0 0\trobot status\t248.746975\t95.565899\t8.481500\t-1.125513\t-0.794605\t153.202888\t0.298000\t-0.001000\n\t\n15:35:51.6\tlog_raw\tgps_raw\t#INSPVAXA,USB3,0,51.0,FINESTEERING,2107,282969.650,02000000,471d,15824;INS_ALIGNMENT_COMPLETE,INS_RTKFIXED,37.37099198077,126.72364195097,8.4825,22.3000,0.1618,-0.2351,-0.0139,-1.127841235,-0.916992124,296.845405459,0.4434,0.2946,0.5560,0.1136,0.0926,0.0774,0.0977,0.1027,4.9114,0f000001,0*282a9ea8\n\tsystem status\tnormal 2 28.000000 0 0\trobot status\t248.625810\t95.641085\t8.482500\t-1.127841\t-0.916992\t153.154595\t0.293000\t-0.005000\n\t\n15:35:52.1\tlog_raw\tgps_raw\t#INSPVAXA,USB3,0,49.5,FINESTEERING,2107,282970.150,02000000,471d,15824;INS_ALIGNMENT_COMPLETE,INS_RTKFIXED,37.37099263807,126.72364060691,8.4830,22.3000,0.1632,-0.2345,-0.0165,-1.327041845,-0.755974067,296.808985126,0.4427,0.2946,0.5559,0.1136,0.0925,0.0774,0.0977,0.1027,4.9120,0f000001,0*fb111f10\n\tsystem status\tnormal 2 28.000000 0 0\trobot status\t248.506755\t95.714039\t8.483000\t-1.327042\t-0.755974\t153.191015\t0.260000\t0.054000\n\t\n15:35:52.6\tlog_raw\tgps_raw\t#INSPVAXA,USB3,0,49.5,FINESTEERING,2107,282970.650,02000000,471d,15824;INS_ALIGNMENT_COMPLETE,INS_RTKFIXED,37.37099330542,126.72363923345,8.4843,22.3000,0.1650,-0.2334,-0.0103,-1.379297675,-0.666693531,296.810188523,0.4427,0.2946,0.5559,0.1136,0.0925,0.0774,0.0977,0.1027,4.9120,0f000001,0*40e7d89f\n\tsystem status\tnormal 2 28.000000 0 0\trobot status\t248.385097\t95.788108\t8.484300\t-1.379298\t-0.666694\t153.189811\t0.256000\t0.066000\n\t\n15:35:53.1\tlog_raw\tgps_raw\t#INSPVAXA,USB3,0,50.5,FINESTEERING,2107,282971.150,02000000,471d,15824;INS_ALIGNMENT_COMPLETE,INS_RTKFIXED,37.37099398804,126.72363786563,8.4853,22.3000,0.1661,-0.2338,-0.0180,-1.270685032,-0.682780948,296.817282496,0.4423,0.2946,0.5559,0.1136,0.0925,0.0774,0.0977,0.1027,4.9128,0f000001,0*f8a30bce\n\tsystem status\tnormal 2 27.900000 0 0\trobot status\t248.263937\t95.863872\t8.485300\t-1.270685\t-0.682781\t153.182718\t0.288000\t0.013000\n\t\n15:35:53.6\tlog_raw\tgps_raw\t#INSPVAXA,USB3,0,50.5,FINESTEERING,2107,282971.650,02000000,471d,15824;INS_ALIGNMENT_COMPLETE,INS_RTKFIXED,37.37099465990,126.72363651456,8.4846,22.3000,0.1699,-0.2362,-0.0068,-1.125018269,-0.570550984,296.760377501,0.4423,0.2946,0.5559,0.1136,0.0925,0.0774,0.0977,0.1027,4.9128,0f000001,0*ee20163a\n\tsystem status\tnormal 2 27.900000 0 0\trobot status\t248.144262\t95.938442\t8.484600\t-1.125018\t-0.570551\t153.239622\t0.292000\t0.006000\n\t\n15:35:54.1\tlog_raw\tgps_raw\t#INSPVAXA,USB3,0,48.5,FINESTEERING,2107,282972.150,02000000,471d,15824;INS_ALIGNMENT_COMPLETE,INS_RTKFIXED,37.37099533114,126.72363514569,8.4846,22.3000,0.1631,-0.2434,-0.0075,-1.229353207,-0.492392608,296.737479032,0.4422,0.2946,0.5560,0.1136,0.0925,0.0774,0.0977,0.1027,4.9138,0f000001,0*e2a3fa7c\n\tsystem status\tnormal 2 28.000000 0 0\trobot status\t248.035923\t96.005381\t8.484600\t-1.202885\t-0.495037\t153.210220\t0.342000\t-0.066000\n\t\n15:35:54.6\tlog_raw\tgps_raw\t#INSPVAXA,USB3,0,48.5,FINESTEERING,2107,282972.650,02000000,471d,15824;INS_ALIGNMENT_COMPLETE,INS_RTKFIXED,37.37099601296,126.72363373726,8.4848,22.3000,0.1655,-0.2434,-0.0062,-1.394785800,-0.542379073,296.812195855,0.4422,0.2946,0.5560,0.1136,0.0925,0.0774,0.0977,0.1027,4.9138,0f000001,0*ee63dd76\n\tsystem status\tnormal 2 28.000000 0 0\trobot status\t247.898253\t96.088618\t8.484800\t-1.394786\t-0.542379\t153.187804\t0.263000\t0.059000\n\t\n15:35:55.1\tlog_raw\tgps_raw\t#INSPVAXA,USB3,0,47.0,FINESTEERING,2107,282973.150,02000000,471d,15824;INS_ALIGNMENT_COMPLETE,INS_RTKFIXED,37.37099670386,126.72363233646,8.4846,22.3000,0.1605,-0.2379,-0.0037,-1.521129756,-0.763571260,296.778124874,0.4424,0.2946,0.5561,0.1137,0.0925,0.0774,0.0977,0.1027,4.9150,0f000001,0*6c9cf6ab\n\tsystem status\tnormal 2 28.000000 0 0\trobot status\t247.774172\t96.165301\t8.484600\t-1.521130\t-0.763571\t153.221875\t0.288000\t0.007000\n\t\n15:35:55.6\tlog_raw\tgps_raw\t#INSPVAXA,USB3,0,47.0,FINESTEERING,2107,282973.650,02000000,471d,15824;INS_ALIGNMENT_COMPLETE,INS_RTKFIXED,37.37099738989,126.72363093033,8.4852,22.3000,0.1673,-0.2327,0.0049,-1.602600322,-0.872352235,296.775722188,0.4424,0.2946,0.5561,0.1137,0.0925,0.0774,0.0977,0.1027,4.9150,0f000001,0*6d258e45\n\tsystem status\tnormal 2 27.900000 0 0\trobot status\t247.649620\t96.241443\t8.485200\t-1.602600\t-0.872352\t153.224278\t0.256000\t0.075000\n\t\n15:35:56.1\tlog_raw\tgps_raw\t\tsystem status\tnormal 2 27.900000 0 0\trobot status\t247.539986\t96.309557\t8.486500\t-1.695799\t-0.929134\t153.191391\t0.262000\t0.062000\n\t\n15:35:56.6\tlog_raw\tgps_raw\t#INSPVAXA,USB3,0,49.0,FINESTEERING,2107,282974.650,02000000,471d,15824;INS_ALIGNMENT_COMPLETE,INS_RTKFIXED,37.37099878397,126.72362813918,8.4887,22.3000,0.1782,-0.2307,0.0009,-1.519938045,-1.116202869,296.818721301,0.4416,0.2946,0.5560,0.1136,0.0925,0.0774,0.0977,0.1027,4.9163,0f000001,0*219b4438\n\tsystem status\tnormal 2 28.000000 0 0\trobot status\t247.402384\t96.396172\t8.488700\t-1.519938\t-1.116203\t153.181279\t0.376000\t-0.114000\n\t\n15:35:57.1\tlog_raw\tgps_raw\t#INSPVAXA,USB3,0,48.5,FINESTEERING,2107,282975.150,02000000,471d,15824;INS_ALIGNMENT_COMPLETE,INS_RTKFIXED,37.37099949137,126.72362674599,8.4896,22.3000,0.1736,-0.2362,0.0047,-1.445494984,-1.113340101,296.818619206,0.4431,0.2948,0.5567,0.1139,0.0926,0.0775,0.0977,0.1028,4.9177,0f000001,0*6f5d7051\n\tsystem status\tnormal 2 28.000000 0 0\trobot status\t247.278978\t96.474686\t8.489600\t-1.445495\t-1.113340\t153.181381\t0.296000\t0.021000\n\t\n15:35:57.6\tlog_raw\tgps_raw\t#INSPVAXA,USB3,0,48.5,FINESTEERING,2107,282975.650,02000000,471d,15824;INS_ALIGNMENT_COMPLETE,INS_RTKFIXED,37.37100019826,126.72362538278,8.4881,22.3000,0.1707,-0.2363,0.0005,-1.379938720,-0.916519890,296.842609438,0.4431,0.2948,0.5567,0.1139,0.0926,0.0775,0.0977,0.1028,4.9177,0f000001,0*5514ce87\n\tsystem status\tnormal 2 28.000000 0 0\trobot status\t247.158227\t96.553144\t8.488100\t-1.379939\t-0.916520\t153.157391\t0.250000\t0.083000\n\t\n15:35:58.1\tlog_raw\tgps_raw\t#INSPVAXA,USB3,0,49.5,FINESTEERING,2107,282976.150,02000000,471d,15824;INS_ALIGNMENT_COMPLETE,INS_RTKFIXED,37.37100091207,126.72362400101,8.4878,22.3000,0.1676,-0.2422,-0.0038,-1.345011262,-0.792526169,296.841980964,0.4425,0.2947,0.5567,0.1137,0.0926,0.0775,0.0977,0.1027,4.9188,0f000001,0*da02f91b\n\tsystem status\tnormal 2 27.900000 0 0\trobot status\t247.035832\t96.632369\t8.487800\t-1.345011\t-0.792526\t153.158019\t0.301000\t0.004000\n\t\n15:35:58.6\tlog_raw\tgps_raw\t#INSPVAXA,USB3,0,49.5,FINESTEERING,2107,282976.650,02000000,471d,15824;INS_ALIGNMENT_COMPLETE,INS_RTKFIXED,37.37100161787,126.72362259542,8.4876,22.3000,0.1713,-0.2361,-0.0000,-1.230290635,-0.956554131,296.705725068,0.4425,0.2947,0.5567,0.1137,0.0926,0.0775,0.0977,0.1027,4.9188,0f000001,0*8e2a3525\n\tsystem status\tnormal 2 27.900000 0 0\trobot status\t246.911327\t96.710706\t8.487600\t-1.230291\t-0.956554\t153.294275\t0.292000\t0.022000\n\t\n15:35:59.1\tlog_raw\tgps_raw\t#INSPVAXA,USB3,0,50.0,FINESTEERING,2107,282977.150,02000000,471d,15824;INS_ALIGNMENT_COMPLETE,INS_RTKFIXED,37.37100231261,126.72362121390,8.4877,22.3000,0.1651,-0.2421,0.0008,-1.098832221,-0.904742170,296.548603231,0.4420,0.2947,0.5566,0.1136,0.0926,0.0774,0.0977,0.1027,4.9199,0f000001,0*083bf95e\n\tsystem status\tnormal 2 27.900000 0 0\trobot status\t246.788954\t96.787815\t8.487700\t-1.098832\t-0.904742\t153.451397\t0.298000\t0.014000\n\t\n15:35:59.6\tlog_raw\tgps_raw\t#INSPVAXA,USB3,0,50.0,FINESTEERING,2107,282977.650,02000000,471d,15824;INS_ALIGNMENT_COMPLETE,INS_RTKFIXED,37.37100299121,126.72361981257,8.4879,22.3000,0.1659,-0.2302,-0.0060,-1.021895005,-0.933563278,296.461558193,0.4420,0.2947,0.5566,0.1136,0.0926,0.0774,0.0977,0.1027,4.9199,0f000001,0*f0f7e65a\n\tsystem status\tnormal 2 27.900000 0 0\trobot status\t246.664827\t96.863133\t8.487900\t-1.021895\t-0.933563\t153.538442\t0.283000\t0.028000\n\t\n15:36:00.1\tlog_raw\tgps_raw\t#INSPVAXA,USB3,0,52.0,FINESTEERING,2107,282978.150,02000000,471d,15824;INS_ALIGNMENT_COMPLETE,INS_RTKFIXED,37.37100367247,126.72361842907,8.4879,22.3000,0.1629,-0.2311,-0.0012,-0.920604944,-1.043526299,296.260165463,0.4427,0.2948,0.5570,0.1137,0.0928,0.0775,0.0977,0.1027,4.9208,0f000001,0*6c36e752\n\tsystem status\tnormal 2 27.900000 0 0\trobot status\t246.542279\t96.938746\t8.487900\t-0.920605\t-1.043526\t153.739835\t0.272000\t0.033000\n\t\n15:36:00.6\tlog_raw\tgps_raw\t#INSPVAXA,USB3,0,52.0,FINESTEERING,2107,282978.650,02000000,471d,15824;INS_ALIGNMENT_COMPLETE,INS_RTKFIXED,37.37100436684,126.72361701359,8.4867,22.3000,0.1639,-0.2335,-0.0162,-0.883856990,-1.214783963,296.168399886,0.4427,0.2948,0.5570,0.1137,0.0928,0.0775,0.0977,0.1027,4.9208,0f000001,0*f7bb67d2\n\tsystem status\tnormal 2 27.900000 0 0\trobot status\t246.416898\t97.015814\t8.486700\t-0.883857\t-1.214784\t153.831600\t0.370000\t-0.102000\n\t\n15:36:01.1\tlog_raw\tgps_raw\t#INSPVAXA,USB3,0,51.5,FINESTEERING,2107,282979.150,02000000,471d,15824;INS_ALIGNMENT_COMPLETE,INS_RTKFIXED,37.37100504962,126.72361562716,8.4847,22.3000,0.1600,-0.2330,-0.0182,-0.879226259,-1.131302419,296.112400832,0.4429,0.2948,0.5572,0.1137,0.0928,0.0775,0.0977,0.1027,4.9212,0f000001,0*44fc000f\n\tsystem status\tnormal 2 28.000000 0 0\trobot status\t246.294090\t97.091595\t8.484700\t-0.879226\t-1.131302\t153.887599\t0.432000\t-0.202000\n\t\n15:36:01.6\tlog_raw\tgps_raw\t\tsystem status\tnormal 2 27.900000 0 0\trobot status\t246.169041\t97.167187\t8.484100\t-0.926329\t-1.223584\t153.988143\t0.213000\t0.127000\n\t\n15:36:02.1\tlog_raw\tgps_raw\t#INSPVAXA,USB3,0,48.0,FINESTEERING,2107,282980.150,02000000,471d,15824;INS_ALIGNMENT_COMPLETE,INS_RTKFIXED,37.37100639827,126.72361280580,8.4843,22.3000,0.1610,-0.2464,-0.0078,-1.128808360,-1.315408116,295.882124797,0.4447,0.2950,0.5582,0.1140,0.0927,0.0775,0.0977,0.1028,4.9213,0f000001,0*5399c86c\n\tsystem status\tnormal 2 27.900000 0 0\trobot status\t246.044179\t97.241282\t8.484300\t-1.128808\t-1.315408\t154.117875\t0.355000\t-0.079000\n\t\n15:36:02.6\tlog_raw\tgps_raw\t#INSPVAXA,USB3,0,48.0,FINESTEERING,2107,282980.650,02000000,471d,15824;INS_ALIGNMENT_COMPLETE,INS_RTKFIXED,37.37100705164,126.72361137761,8.4834,22.3000,0.1707,-0.2402,-0.0119,-1.407160941,-1.329354223,295.708309677,0.4447,0.2950,0.5582,0.1140,0.0927,0.0775,0.0977,0.1028,4.9213,0f000001,0*d4834280\n\tsystem status\tnormal 2 27.900000 0 0\trobot status\t245.917672\t97.313800\t8.483400\t-1.407161\t-1.329354\t154.291690\t0.263000\t0.067000\n\t\n15:36:03.1\tlog_raw\tgps_raw\t#INSPVAXA,USB3,0,48.5,FINESTEERING,2107,282981.150,02000000,471d,15824;INS_ALIGNMENT_COMPLETE,INS_RTKFIXED,37.37100772173,126.72360998460,8.4814,22.3000,0.1860,-0.2371,-0.0157,-1.203417733,-1.261430362,295.578766556,0.4455,0.2951,0.5589,0.1141,0.0926,0.0776,0.0977,0.1028,4.9213,0f000001,0*2091f446\n\tsystem status\tnormal 2 27.900000 0 0\trobot status\t245.794281\t97.388173\t8.481400\t-1.203418\t-1.261430\t154.421233\t0.264000\t0.066000\n\t\n15:36:03.6\tlog_raw\tgps_raw\t\tsystem status\tnormal 2 27.900000 0 0\trobot status\t245.671083\t97.462988\t8.476500\t-0.879247\t-1.278490\t154.524074\t0.350000\t-0.056000\n\t\n15:36:04.1\tlog_raw\tgps_raw\t\tsystem status\tnormal 2 27.900000 0 0\trobot status\t245.548324\t97.535797\t8.471000\t-0.912734\t-1.315304\t154.588410\t0.258000\t0.074000\n\t\n15:36:04.6\tlog_raw\tgps_raw\t\tsystem status\tnormal 2 27.900000 0 0\trobot status\t245.424899\t97.608212\t8.466300\t-1.011673\t-1.263689\t154.596842\t0.326000\t-0.041000\n\t\n15:36:05.1\tlog_raw\tgps_raw\t#INSPVAXA,USB3,0,51.0,FINESTEERING,2107,282983.150,02000000,471d,15824;INS_ALIGNMENT_COMPLETE,INS_RTKFIXED,37.37101036366,126.72360442489,8.4628,22.3000,0.1755,-0.2357,-0.0080,-1.025739547,-1.189368406,295.388361945,0.4463,0.2951,0.5596,0.1141,0.0926,0.0776,0.0978,0.1028,4.9221,0f000001,0*2959208b\n\tsystem status\tnormal 2 27.900000 0 0\trobot status\t245.301811\t97.681401\t8.462800\t-1.025740\t-1.189368\t154.611638\t0.284000\t0.031000\n\t\n15:36:05.6\tlog_raw\tgps_raw\t#INSPVAXA,USB3,0,51.0,FINESTEERING,2107,282983.650,02000000,471d,15824;INS_ALIGNMENT_COMPLETE,INS_RTKFIXED,37.37101102324,126.72360304881,8.4600,22.3000,0.1712,-0.2258,-0.0116,-0.859579681,-1.039097489,295.288660935,0.4463,0.2951,0.5596,0.1141,0.0926,0.0776,0.0978,0.1028,4.9221,0f000001,0*ad7af1a9\n\tsystem status\tnormal 2 28.000000 0 0\trobot status\t245.179920\t97.754608\t8.460000\t-0.859580\t-1.039097\t154.711339\t0.281000\t0.027000\n\t\n15:36:06.1\tlog_raw\tgps_raw\t#INSPVAXA,USB3,0,50.5,FINESTEERING,2107,282984.150,02008000,471d,15824;INS_ALIGNMENT_COMPLETE,INS_RTKFIXED,37.37101166488,126.72360167491,8.4566,22.3000,0.1754,-0.2281,-0.0207,-0.961299584,-0.781860574,295.230299277,0.4466,0.2950,0.5599,0.1142,0.0925,0.0776,0.0978,0.1028,4.9229,0f000001,0*2cbfc422\n\tsystem status\tnormal 2 27.900000 0 0\trobot status\t245.058223\t97.825824\t8.456600\t-0.961300\t-0.781861\t154.769701\t0.296000\t0.009000\n\t\n15:36:06.6\tlog_raw\tgps_raw\t\tsystem status\tnormal 2 28.000000 0 0\trobot status\t244.937880\t97.895786\t8.454100\t-0.986638\t-0.509016\t154.801608\t0.358000\t-0.093000\n\t\n15:36:07.1\tlog_raw\tgps_raw\t#INSPVAXA,USB3,0,46.0,FINESTEERING,2107,282985.150,02008000,471d,15824;INS_ALIGNMENT_COMPLETE,INS_RTKFIXED,37.37101294073,126.72359895253,8.4524,22.3000,0.1696,-0.2376,-0.0054,-0.854565815,-0.366619104,295.159142315,0.4467,0.2950,0.5599,0.1143,0.0926,0.0776,0.0978,0.1028,4.9242,0f000001,0*a94814eb\n\tsystem status\tnormal 2 28.000000 0 0\trobot status\t244.817079\t97.967431\t8.452400\t-0.854566\t-0.366619\t154.840858\t0.260000\t0.057000\n\t\n15:36:07.6\tlog_raw\tgps_raw\t#INSPVAXA,USB3,0,46.0,FINESTEERING,2107,282985.650,02008000,471d,15824;INS_ALIGNMENT_COMPLETE,INS_RTKFIXED,37.37101359136,126.72359755019,8.4503,22.3000,0.1680,-0.2437,-0.0157,-0.803804661,-0.502558693,295.184613052,0.4467,0.2950,0.5599,0.1143,0.0926,0.0776,0.0978,0.1028,4.9242,0f000001,0*db0a5a5c\n\tsystem status\t
